vi "HMI.vi"(5 "Disabled":bool=TRUE, 8 "HMI to Control":T1={"RightDriveValue"=0.0, "LeftDriveValue"=0.0, "Intake Value"=0.0, "Shooter States"=enum."Shooter Off", "Collector Lift States"=enum."Collector Manual", "Shooter Hood States"=enum."Hood Close Shot", "Fire "=FALSE, "Collector Lift Manual Value"=0.0, "Shooter Hood Manual Value"=0.0, " Autolift portcullis"=FALSE, "Autoadjust CDF"=FALSE, "Hood Manual Request"=FALSE, "Collect Lift Manual Request"=FALSE, "Keep at target "=FALSE, "Hood Manual No."=0, "Collect Lift Manual No. "=0}, 9 "Gamepad Data":T5) -> (2 "HMI to Control":T1={"RightDriveValue"=0.0, "LeftDriveValue"=0.0, "Intake Value"=0.0, "Shooter States"=enum."Shooter Off", "Collector Lift States"=enum."Collector Manual", "Shooter Hood States"=enum."Hood Close Shot", "Fire "=FALSE, "Collector Lift Manual Value"=0.0, "Shooter Hood Manual Value"=0.0, " Autolift portcullis"=FALSE, "Autoadjust CDF"=FALSE, "Hood Manual Request"=FALSE, "Collect Lift Manual Request"=FALSE, "Keep at target "=FALSE, "Hood Manual No."=0, "Collect Lift Manual No. "=0}, 3 "Gamepad Data Out":T5)   [LabVIEW 2015]
uses:
  Typedefs/GamepadData.ctl
  Typedefs/HMI_to_Control.ctl
  Typedefs/Shooter States.ctl
  Typedefs/CollectorLiftStates.ctl
  Typedefs/Hood States.ctl
  Auton/scriptlib/auto_data.vi
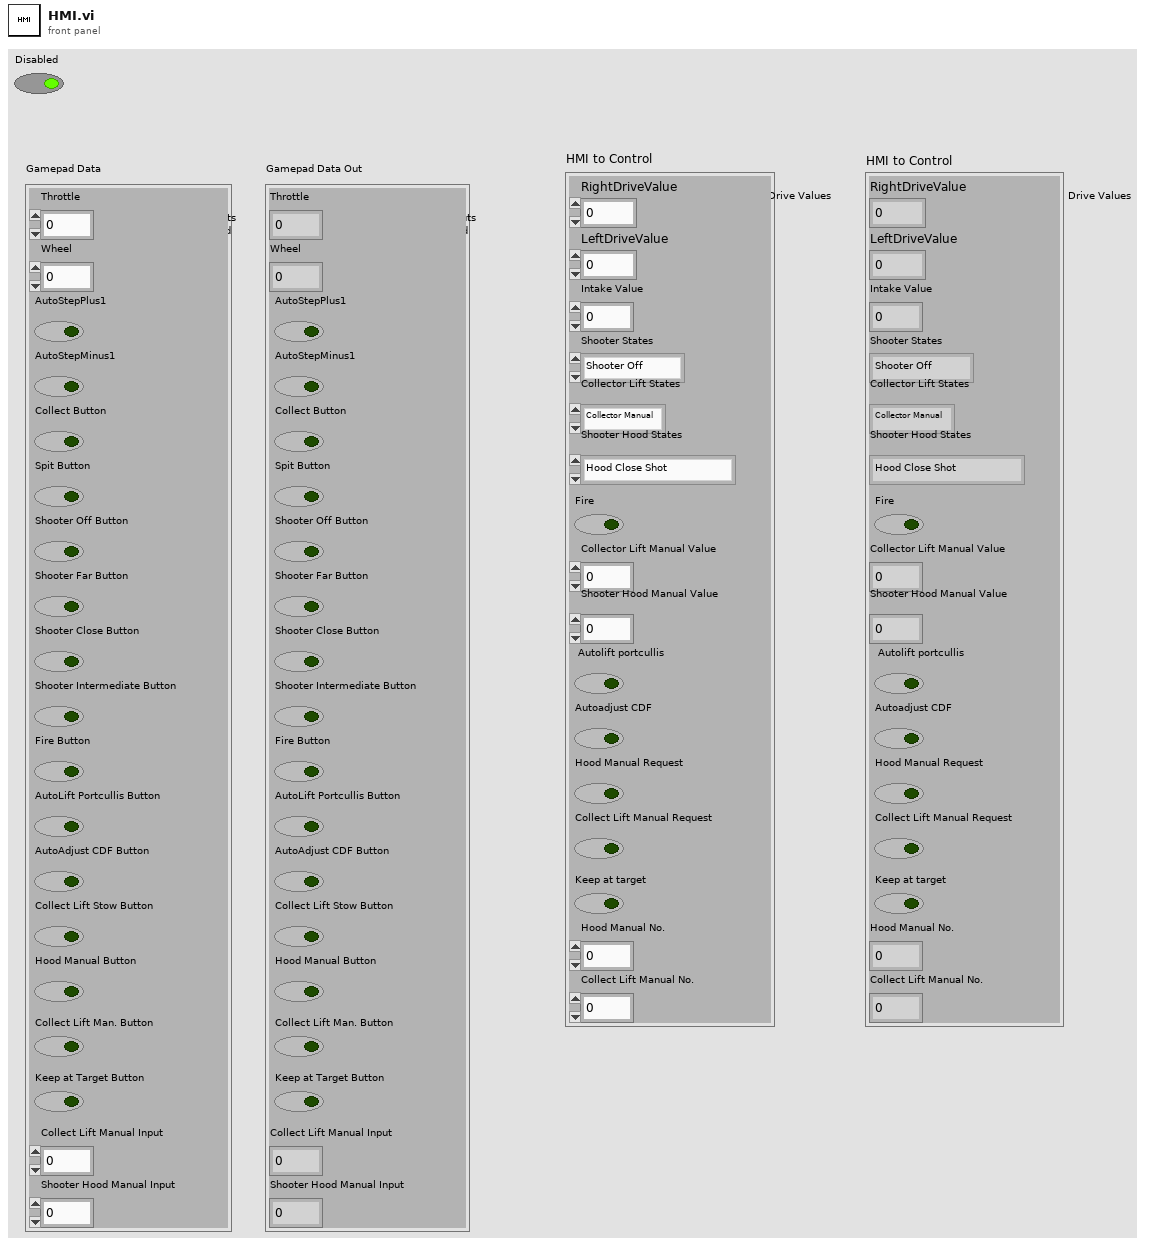
[diagram p1: front panel]
types:
  T1 = typedef "HMI_to_Control.ctl" = cluster{"RightDriveValue":dbl, "LeftDriveValue":dbl, "Intake Value":dbl, "Shooter States":T2, "Collector Lift States":T3, "Shooter Hood States":T4, "Fire ":bool, "Collector Lift Manual Value":dbl, "Shooter Hood Manual Value":dbl, " Autolift portcullis":bool, "Autoadjust CDF":bool, "Hood Manual Request":bool, "Collect Lift Manual Request":bool, "Keep at target ":bool, "Hood Manual No.":i8, "Collect Lift Manual No. ":i8}
  T2 = typedef "Shooter States.ctl" = enum16{"Shooter Off", "Shooter Far", "Shooter Close", "Shooter Intermediate", "Shooter Spy"}
  T3 = typedef "CollectorLiftStates.ctl" = enum16{"Collector Manual", "Stow", "Collect Position", "Spit Position", "Portcullis Set Up", "Portcullis Lift Up", "CDF Set Up", "Push CDF Down"}
  T4 = typedef "Hood States.ctl" = enum16{"Hood Manual ", "Hood Close Shot", "Hood Far Shot", "Hood Spy Shot", "Hood Intermediate"}
  T5 = typedef "GamepadData.ctl" = cluster{"Throttle":dbl, "Wheel":dbl, "AutoStepPlus1":bool, "AutoStepMinus1":bool, "Collect Button":bool, "Spit Button":bool, "Shooter Off Button":bool, "Shooter Far Button":bool, "Shooter Close Button":bool, "Shooter Intermediate Button":bool, "Fire Button":bool, "AutoLift Portcullis Button":bool, "AutoAdjust CDF Button":bool, "Collect Lift Stow Button":bool, "Hood Manual Button":bool, "Collect Lift Man. Button":bool, "Keep at Target Button":bool, "Collect Lift Manual Input":dbl, "Shooter Hood Manual Input":dbl}
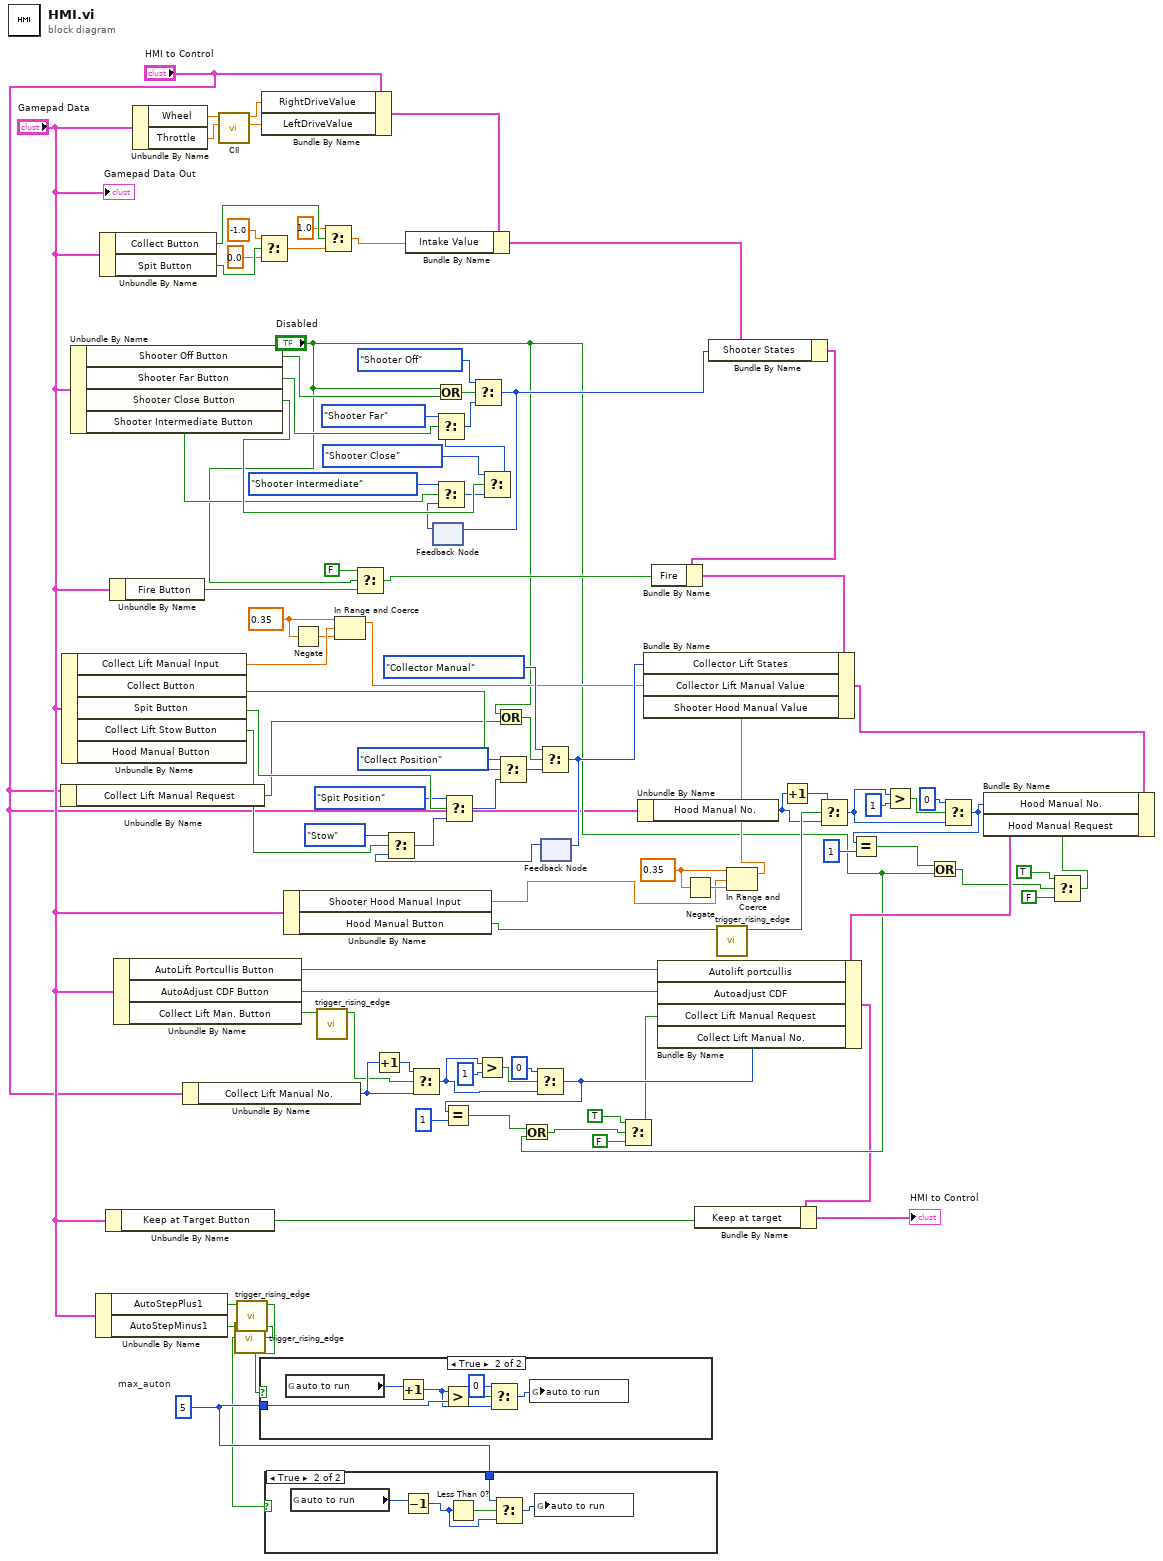
[diagram p0: block diagram]
diagram:
  w45 = 0.35 ("upper limit")
  w47 = 0.35 ("upper limit")
  w95 = i8 5  # max_auton
  n1 = Unbundle By Name("HMI to Control") -> ("Collect Lift Manual Request"=w3:bool)
  n2 = Unbundle By Name("Gamepad Data") -> ("Collect Lift Manual Input"=w48:dbl, "Collect Button"=w59:bool, "Spit Button"=w57:bool, "Collect Lift Stow Button"=w52:bool)  [unwired: 1 out]
  n3 = Unbundle By Name("Gamepad Data") -> ("Shooter Off Button"=w81:bool, "Shooter Far Button"=w77:bool, "Shooter Close Button"=w76:bool, "Shooter Intermediate Button"=w65:bool)
  n4 = Unbundle By Name("Gamepad Data") -> ("AutoStepPlus1"=w94:bool, "AutoStepMinus1"=w92:bool)
  n5 = Unbundle By Name("Gamepad Data") -> ("Collect Button"=w89:bool, "Spit Button"=w87:bool)
  n6 = Unbundle By Name("Gamepad Data") -> ("Keep at Target Button"=w5:bool)
  n7 = Unbundle By Name("Gamepad Data") -> ("Fire Button"=w70:bool)
  n8 = Unbundle By Name("Gamepad Data") -> ("AutoLift Portcullis Button"=w42:bool, "AutoAdjust CDF Button"=w41:bool, "Collect Lift Man. Button"=w9:bool)
  n9 = Unbundle By Name("Gamepad Data") -> ("Wheel"=w99:dbl, "Throttle"=w98:dbl)
  n10 = Unbundle By Name("HMI to Control") -> ("Collect Lift Manual No."=w16:i8)
  n11 = call "CII.vi"("Wheel"=w99, "Throttle"=w98) -> ("RightDrive"=w97:dbl, "LeftDrive"=w96:dbl)  [unwired: 7 in]
  n12 = call "trigger_rising_edge.vi"("input"=w92) -> ("rising"=w91:bool)  [unwired: 10 in]
  n13 = call "trigger_rising_edge.vi"("input"=w94) -> ("rising"=w93:bool)  [unwired: 10 in]
  n14 = Select(t=-1.0, s=w87, f=0.0) -> (s? t:f=w85:dbl)
  n15 = case shown="True" w93 {
    tunnel: w95 -> [_ w103]
    frame False {
    }
    frame True {
      n16 = global read "auto_data.vi" "auto to run"() -> (w105:i8)
      n17 = Increment(x=w105) -> (x+1=w102:i8)
      n18 = Greater?(x=w102, y=w103) -> (0:w104:bool)
      n19 = Select(t=i8 0, s=w104, f=w102) -> (s? t:f=w100:i8)
      n20 = global write "auto_data.vi" "auto to run"(w100) -> ()
    }
  }
  n21 = Bundle By Name(cluster="HMI to Control", "RightDriveValue"=w97, "LeftDriveValue"=w96) -> (w90:T1)
  n22 = case shown="True" w91 {
    tunnel: w95 -> [_ w107]
    frame False {
    }
    frame True {
      n23 = global read "auto_data.vi" "auto to run"() -> (w110:i8)
      n24 = Decrement(x=w110) -> (x-1=w106:i8)
      n25 = Less Than 0?(x=w106) -> (x < 0?=w109:bool)
      n26 = Select(t=w107, s=w109, f=w106) -> (s? t:f=w108:i8)
      n27 = global write "auto_data.vi" "auto to run"(w108) -> ()
    }
  }
  n28 = Unbundle By Name("Gamepad Data") -> ("Shooter Hood Manual Input"=w40:dbl, "Hood Manual Button"=w30:bool)
  n29 = Negate(x=w47) -> (-x=w46:dbl)
  n30 = call "trigger_rising_edge.vi"("input"=w9) -> ("rising"=w2:bool)  [unwired: 10 in]
  n31 = Select(t=1.0, s=w89, f=w85) -> (s? t:f=w84:dbl)
  n32 = In Range and Coerce(upper limit=w47, x=w48, lower limit=w46) -> (coerced(x)=w49:dbl)  [unwired: 1 out]
  n33 = Select(t=FALSE, s="Disabled", f=w70) -> (s? t:f=w68:bool)
  n34 = Increment(x=w16) -> (x+1=w17:i8)
  n35 = Bundle By Name(cluster=w90, "Intake Value"=w84) -> (w74:T1)
  n36 = Select(t=w17, s=w2, f=w16) -> (s? t:f=w15:i8)
  n37 = feedback #1() -> (w67:T2)  [unwired: 1 in]
  n38 = Or(x="Disabled", y=w81) -> (x .or. y?=w80:bool)
  n39 = Select(t=Shooter_States."Shooter Intermediate", s=w65, f=w67) -> (s? t:f=w64:T2)
  n40 = Greater?(x=w15, y=i8 1) -> (0:w21:bool)
  n41 = Select(t=Shooter_States."Shooter Close", s=w76, f=w64) -> (s? t:f=w73:T2)
  n42 = Select(t=Shooter_States."Shooter Far" ("Enum"), s=w77, f=w73) -> (s? t:f=w78:T2)
  n43 = Select(t=Shooter_States."Shooter Off" ("Enum"), s=w80, f=w78) -> (s? t:f=w72:T2)
  n44 = feedback-in #1(w72) -> ()
  n45 = Or(x="Disabled", y=w3) -> (x .or. y?=w63:bool)
  n46 = Select(t=i8 0, s=w21, f=w15) -> (s? t:f=w14:i8)
  n47 = Equal?(x=w14, y=i8 1) -> (x = y?=w18:bool)
  n48 = Or(x=w18, y="Disabled") -> (x .or. y?=w1:bool)
  n49 = feedback #2() -> (w50:T3)  [unwired: 1 in]
  n50 = Select(t=CollectorLiftStates."Stow" ("Collector Lift States"), s=w52, f=w50) -> (s? t:f=w53:T3)
  n51 = Select(t=CollectorLiftStates."Spit Position" ("Collector Lift States"), s=w57, f=w53) -> (s? t:f=w55:T3)
  n52 = Select(t=CollectorLiftStates."Collect Position" ("Collector Lift States"), s=w59, f=w55) -> (s? t:f=w58:T3)
  n53 = Select(t=CollectorLiftStates."Collector Manual" ("Collector Lift States"), s=w63, f=w58) -> (s? t:f=w51:T3)
  n54 = feedback-in #2(w51) -> ()
  n55 = Select(t=TRUE, s=w1, f=FALSE) -> (s? t:f=w10:bool)
  n56 = Unbundle By Name("HMI to Control") -> ("Hood Manual No."=w32:i8)
  n57 = Negate(x=w45) -> (-x=w44:dbl)
  n58 = Bundle By Name(cluster=w74, "Shooter States"=w72) -> (w71:T1)
  n59 = Bundle By Name(cluster=w71, "Fire"=w68) -> (w61:T1)
  n60 = call "trigger_rising_edge.vi"("input"=w30) -> ("rising"=w33:bool)  [unwired: 10 in]
  n61 = In Range and Coerce(upper limit=w45, x=w40, lower limit=w44) -> (coerced(x)=w43:dbl)  [unwired: 1 out]
  n62 = Bundle By Name(cluster=w61, "Collector Lift States"=w51, "Collector Lift Manual Value"=w49, "Shooter Hood Manual Value"=w43) -> (w39:T1)
  n63 = Increment(x=w32) -> (x+1=w34:i8)
  n64 = Select(t=w34, s=w33, f=w32) -> (s? t:f=w31:i8)
  n65 = Greater?(x=w31, y=i8 1) -> (0:w36:bool)
  n66 = Select(t=i8 0, s=w36, f=w31) -> (s? t:f=w28:i8)
  n67 = Equal?(x=w28, y=i8 1) -> (x = y?=w24:bool)
  n68 = Or(x=w24, y="Disabled") -> (x .or. y?=w23:bool)
  n69 = Select(t=TRUE, s=w23, f=FALSE) -> (s? t:f=w25:bool)
  n70 = Bundle By Name(cluster=w39, "Hood Manual No."=w28, "Hood Manual Request"=w25) -> (w38:T1)
  n71 = Bundle By Name(cluster=w38, "Autolift portcullis"=w42, "Autoadjust CDF"=w41, "Collect Lift Manual Request"=w10, "Collect Lift Manual No."=w14) -> (w7:T1)
  n72 = Bundle By Name(cluster=w7, "Keep at target"=w5) -> (→"HMI to Control":T1)
  "Gamepad Data Out" <- "Gamepad Data"
